vi "Actor Core.vi"(8 "error in":errorcluster, 11 "ATM Controller in":refnum<class "ATM Controller.lvclass">) -> (0 "error out":errorcluster, 3 "Actor out":refnum<class "Actor.lvclass">)   [LabVIEW 2019, in "ATM Controller.lvlib" / "ATM Controller.lvclass"]
doc: "(<B>Filename</B>: Actor Framework.lvlib:Actor.lvclass:Actor Core.vi)\n\nReceives messages to the actor, reacts to them, and initiates any error handling that may shut the actor down.\n\nDescendant classes may override this VI to append parallel tasks for the actor to complete while it handles messages. Overrides use the Call Parent Method node."
uses:
  ATM Controller.lvclass
  <vilib>/ActorFramework/Stop Msg/Stop Msg.lvclass
  <vilib>/ActorFramework/Actor/Actor.lvclass
  C:/Program Files (x86)/National Instruments/LabVIEW 2019/vi.lib/ActorFramework/Actor/Actor.lvclass
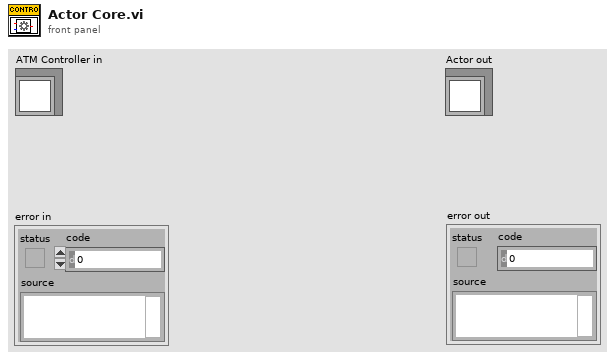
[diagram p1: front panel]
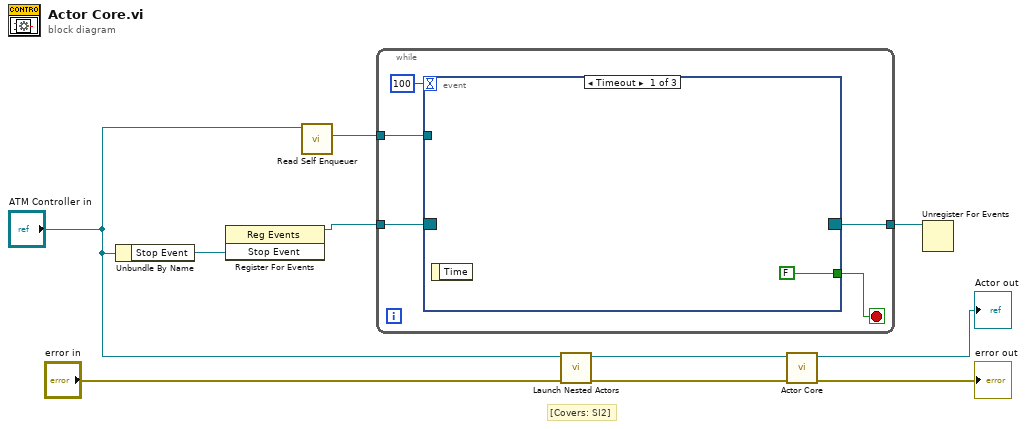
[diagram p0: block diagram]
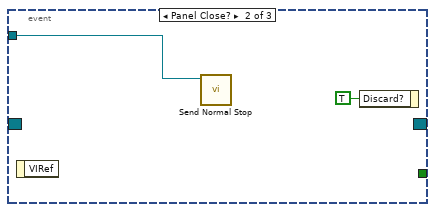
[diagram p2: hidden frame]
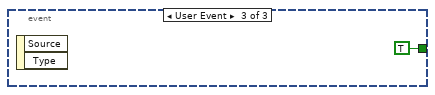
[diagram p3: hidden frame]
diagram:
  # "[Covers: SI2]"
  n1 = Unbundle By Name("ATM Controller in") -> ("Stop Event"=w2:refnum<user-event>)
  n2 = register-events(w2) -> (reference out=w5:refnum<event-registration>)  [unwired: 2 in, 1 out]
  n3 = call <vilib>:"Read Self Enqueuer.vi"("Actor"="ATM Controller in") -> ("Self Enqueuer"=w3:refnum<class "Message Enqueuer.lvclass">)  [unwired: 10 in]
  n4 = while {
    tunnel: w5 -> [w14]
    tunnel: [w13] -> w4
    tunnel: w3 -> [w12]
    stop <- w15 stop-if-true
    n5 = event shown="[0] Timeout" {
      selector: w14 -> [_ _ _]
      dyn-events: [_ _ _] -> w13
      timeout: 100 -> [_ _ _]
      tunnel: [FALSE _ TRUE] -> w15
      tunnel: w12 -> [_ w17 _]
      event Timeout {
        n6 = event-data() -> ()  [unwired: 1 in, 1 out]
      }
      event Panel Close? {
        n7 = event-data() -> ()  [unwired: 1 in, 1 out]
        n8 = call <vilib>:"Send Normal Stop.vi"("Message Enqueuer"=w17) -> ()  [unwired: 10 in, 1 out]
        n9 = event-data("Discard?"=TRUE) -> ()  [unwired: 1 in, 1 out]
      }
      event User Event {
        n10 = event-data() -> ()  [unwired: 1 in, 2 out]
      }
    }
  }
  n11 = call "Launch Nested Actors.vi"("error in (no error)"="error in", "ATM Controller in"="ATM Controller in") -> ("error out"=w7:errorcluster, "ATM Controller out"=w6:refnum<class "ATM Controller.lvclass">)  [unwired: 8 in]
  n12 = call-parent "Actor Core.vi"("error in"=w7, "Actor in"=w6) -> ("error out"=→"error out":errorcluster, "Actor out"=→"Actor out":refnum<class "Actor.lvclass">)  [unwired: 8 in]
  n13 = Unregister For Events(event registration refnum=w4) -> ()  [unwired: 1 in, 1 out]
